vi "Main Tclk.vi"() -> ()   [LabVIEW 2018] (continued)
                          "PID recovered" <- TRUE
                        }
                      }
                    }
                    frame True {
                      w5810 = FALSE
                      n1350 = Divide(x=w5823, y=w5822) -> (x/y=w5821:dbl)
                      n1351 = expression code="x/100"("PID Target (%)") -> (w5816:sgl)
                      n1352 = local write "PID recovered"(w5810) -> ()
                      n1353 = Subtract(x=sgl 1.0, y=w5816) -> (x-y=w5817:sgl)
                      n1354 = Multiply(x=w5821, y=w5817) -> (x*y=w5820:dbl)
                      n1355 = Add(x=w5820, y=w5816) -> (x+y=w5818:dbl)
                      n1356 = Multiply(x=w5818, y=w5811) -> (x*y=w5814:dbl)
                      n1357 = Bundle By Name(cluster=w5812, "FIB PID target"=w5814) -> (w5813:T35)
                      n1358 = local write "Milling para"(w5813) -> ()
                      "Run once" <- w5810
                    }
                  }
                  n1359 = case shown="True" w5786 {
                    frame False {
                    }
                    frame True {
                      n1360 = stacked-sequence {
                        seq-local: [_ w5825 _] -> [_ _ w5860]
                        frame #0 {
                          n1361 = Wait (ms)(milliseconds to wait=u32 2000) -> ()  [unwired: 1 out]
                        }
                        frame #1 {
                          n1362 = local read "Machine Type"() -> (w5826:u8)
                          n1363 = case shown="2" w5826 {
                            tunnel: [w5827 w5835] -> w5825
                            frame 0, Default {
                              n1364 = local read "HV Data Output"() -> (w5831:T18)
                              n1365 = local read "Reheat Parameters"() -> (w5832:T1)
                              n1366 = Unbundle By Name(w5831) -> ("Emission (uA)"=w5833:sgl)
                              n1367 = Unbundle By Name(w5832) -> ("Emission (uA)"=w5834:sgl)
                              n1368 = Subtract(x=w5833, y=w5834) -> (x-y=w5828:sgl)
                              n1369 = Absolute Value(x=w5828) -> (abs(x)=w5829:sgl)
                              n1370 = Greater?(x=0.1 ("y"), y=w5829) -> (0:w5827:bool)
                            }
                            frame 2 {
                              n1371 = stacked-sequence {
                                tunnel: [_ w5859] -> w5835
                                frame #0 {
                                n1372 = local read "FIB HV target matched"() -> (w5837:bool)
                                n1373 = And(x="FIB probe auto min", y=w5837) -> (x .and. y?=w5838:bool)
                                n1374 = case shown="True" w5838 {
                                frame False {
                                }
                                frame True {
                                n1375 = local read "Api"() -> (w5842:refnum<k7>)
                                n1376 = local read "FIB Milling Probe"() -> (w5840:string)
                                n1377 = call "SmartSEM Remote API goto min or max FIB probe current.vi"("Min or Max"="Min", "FIB Probe"=w5840, "Api"=w5842) -> ("Goto probe"=w5841:string)  [unwired: 7 in, 1 out]
                                n1378 = local write "FIB Milling Probe"(w5841) -> ()
                                }
                                }
                                }
                                frame #1 {
                                n1379 = local read "Api"() -> (w5843:refnum<k7>)
                                n1380 = local read "FIB Parameters"() -> (w5858:T19)
                                n1381 = call "SmartSEM Remote API FIB Faraday cup.vi"("Api"=w5843) -> ("FIB Faraday Cup (nA)"=w5856:sgl)  [unwired: 8 in, 2 out]
                                n1382 = call "SmartSEM Remote API get FIB HV data.vi"("Api in"=w5843) -> ("Capella HV Data Output"=w5845:T17)  [unwired: 7 in, 3 out]
                                n1383 = Unbundle By Name(w5858) -> ("FIB probe current"=w5857:sgl)
                                n1384 = Unbundle By Name(w5845) -> ("Emission Target (uA)"=w5847:sgl, "Emission Actual (uA)"=w5846:sgl)
                                n1385 = local read "FIB HV target matched"() -> (w5851:bool)
                                n1386 = Divide(x=w5856, y=w5857) -> (x/y=w5855:sgl)
                                n1387 = Subtract(x=w5847, y=w5846) -> (x-y=w5850:sgl)
                                n1388 = Absolute Value(x=w5850) -> (abs(x)=w5849:sgl)
                                n1389 = In Range and Coerce(upper limit=sgl 1.5 ("y"), x=w5855, lower limit=sgl 0.8 ("y")) -> (In Range?=w5852:bool)  [unwired: 1 out]
                                n1390 = Less?(x=w5849, y=sgl 0.1) -> (x < y?=w5844:bool)
                                n1391 = Compound Arithmetic op=AND(w5851, w5852, w5844) -> (w5859:bool)
                                }
                              }
                            }
                          }
                        }
                        frame #2 {
                          n1392 = case shown="True" w5860 {
                            frame False {
                            }
                            frame True {
                              n1393 = stacked-sequence {
                                frame #0 {
                                w5861 = dbl[] [] ("Re-engage Delta X array")
                                w5862 = 0.0 ("Re-engage X shift")
                                n1394 = local write "Re-engage X shift (um)"(w5862) -> ()
                                n1395 = local write "Re-engage Y shift (um)"(w5862) -> ()
                                n1396 = local write "Re-engage Delta X array"(w5861) -> ()
                                n1397 = local write "Re-engage Delta Y array"(w5861) -> ()
                                n1398 = local write "Re-engage X shift array"(w5861) -> ()
                                n1399 = local write "Re-engage Y shift array"(w5861) -> ()
                                }
                                frame #1 {
                                n1400 = local read "Machine Type"() -> (w5864:u8)
                                n1401 = case shown="2" w5864 {
                                tunnel: [w5865 w5873 w5874] -> w5863
                                frame 0, Default {
                                n1402 = for {
                                N: 10 -> [_]
                                tunnel: [w5870] -> w5867 mode=indexing
                                n1403 = shared-variable ".\\Zeiss Library.lvlib\\Logs"() -> (w5872:sgl[])  [unwired: 1 in, 1 out]
                                n1404 = Index Array(array=w5872, index=0) -> (element=w5870:sgl)
                                n1405 = Wait Until Next ms Multiple(millisecond multiple=u32 10) -> ()  [unwired: 1 out]
                                }
                                n1406 = call-poly <vilib>:"Basic Averaged DC-RMS.vi"("signal in"=w5867) -> ("DC value"=w5866:dbl)  [unwired: 7 in, 3 out]
                                n1407 = To Single Precision Float(number=w5866) -> (single precision float=w5865:sgl)
                                }
                                frame 1 {
                                n1408 = local read "Faraday Cup (nA)"() -> (w5873:sgl)
                                }
                                frame 2 {
                                n1409 = for {
                                N: 10 -> [_]
                                tunnel: [w5879] -> w5876 mode=indexing
                                n1410 = shared-variable ".\\Zeiss Library.lvlib\\Logs"() -> (w5881:sgl[])  [unwired: 1 in, 1 out]
                                n1411 = Index Array(array=w5881, index=0) -> (element=w5879:sgl)
                                n1412 = Wait Until Next ms Multiple(millisecond multiple=u32 10) -> ()  [unwired: 1 out]
                                }
                                n1413 = call-poly <vilib>:"Basic Averaged DC-RMS.vi"("signal in"=w5876) -> ("DC value"=w5875:dbl)  [unwired: 7 in, 3 out]
                                n1414 = To Single Precision Float(number=w5875) -> (single precision float=w5874:sgl)
                                }
                                }
                                n1415 = shared-variable ".\\Zeiss Library.lvlib\\Faraday Cup before mill"(w5863) -> ()  [unwired: 1 in, 1 out]
                                n1416 = local write "Faraday Cup before mill"(w5863) -> ()
                                }
                                frame #2 {
                                w5882 = u8 0 ("Re-engage counts")
                                w5883 = FALSE ("Reheat")
                                n1417 = local write "Re-engage counts"(w5882) -> ()
                                n1418 = local write "Recovered counts"(w5882) -> ()
                                n1419 = local write "Last re-engage count"(w5882) -> ()
                                n1420 = local write "Pause for reheat"(w5883) -> ()
                                n1421 = local write "Mill Manual Pause"(w5883) -> ()
                                n1422 = local write "Reheat from last"(w5883) -> ()
                                }
                                frame #3 {
                                w5885 = TRUE ("Reset WD")
                                n1423 = local read "Alert Settings"() -> (w5884:T36)
                                n1424 = local write "SW error warning armed"(w5885) -> ()
                                n1425 = local write "Auto re-engage"(w5885) -> ()
                                n1426 = local write "3D image paused armed"(w5885) -> ()
                                n1427 = local write "Temperature warning armed"(w5885) -> ()
                                n1428 = local write "Prior Alert Settings"(w5884) -> ()
                                }
                                frame #4 {
                                n1429 = Get Date/Time In Seconds() -> (seconds since 1Jan1904=w5886:timestamp)
                                n1430 = local write "Auto reheat running"(FALSE ("Auto reheat running")) -> ()
                                n1431 = local write "Re-engage time"(w5886) -> ()
                                n1432 = property on="Mill Manual Pause" class="Bool (strict)"("DisabledEnum"=T44."Enabled" ("Disabled")) -> ()  [unwired: 2 in, 2 out]
                                }
                              }
                            }
                          }
                        }
                      }
                    }
                  }
                  n1433 = Compound Arithmetic op=OR(w5790, w5789, w5795) -> (w5796:bool)
                }
                n1434 = case shown="True" w5766 {
                  frame False {
                  }
                  frame True {
                    w5769 = T44."Enabled" ("Disabled")
                    n1435 = property on="Scan x1" class="Bool (strict)"("DisabledEnum"=w5769) -> ()  [unwired: 2 in, 2 out]
                    n1436 = property on="Scan xn" class="Bool (strict)"("DisabledEnum"=w5769) -> ()  [unwired: 2 in, 2 out]
                    n1437 = property on="Start Current DataLog" class="Bool (strict)"("DisabledEnum"=w5769) -> ()  [unwired: 2 in, 2 out]
                    n1438 = property on="Pre image" class="Bool (strict)"("DisabledEnum"=w5769) -> ()  [unwired: 2 in, 2 out]
                    n1439 = property on="Post image" class="Bool (strict)"("DisabledEnum"=w5769) -> ()  [unwired: 2 in, 2 out]
                    n1440 = property on="FIB Imaging" class="Bool (strict)"("DisabledEnum"=w5769) -> ()  [unwired: 2 in, 2 out]
                    n1441 = property on="FIB time lapse" class="Bool (strict)"("DisabledEnum"=w5769) -> ()  [unwired: 2 in, 2 out]
                    n1442 = property on="Reset" class="Bool (strict)"("DisabledEnum"=w5769) -> ()  [unwired: 2 in, 2 out]
                  }
                }
                n1443 = Or(x=w5767, y=w5766) -> (x .or. y?=w5765:bool)
                n1444 = shared-variable "My Computer\\Zeiss Library.lvlib\\Milling Stop"(w5765) -> ()  [unwired: 1 in, 1 out]
                n1445 = shared-variable "My Computer\\Zeiss Library.lvlib\\Milling Resume"(FALSE ("Milling Resume")) -> ()  [unwired: 1 in, 1 out]
              }
              frame #8 {
                w5966 = sgl 0.0 ("Single")
                n1446 = shared-variable ".\\Zeiss Library.lvlib\\Specimen (nA)"() -> (→"Specimen I (nA)":sgl)  [unwired: 1 in, 1 out]
                n1447 = shared-variable ".\\Zeiss Library.lvlib\\Beam Dump 1 (nA)"() -> (→"Beam Dump 1 (nA)":sgl)  [unwired: 1 in, 1 out]
                n1448 = shared-variable ".\\Zeiss Library.lvlib\\Beam Dump 2 (nA)"() -> (→"Beam Dump 2 (nA)":sgl)  [unwired: 1 in, 1 out]
                n1449 = shared-variable ".\\Zeiss Library.lvlib\\Milling I (nA)"() -> (→"Milling I (nA)":sgl)  [unwired: 1 in, 1 out]
                n1450 = shared-variable ".\\Zeiss Library.lvlib\\Milling Z Voltage"() -> (w5947:sgl)  [unwired: 1 in, 1 out]
                "Milling Z voltage (V)" <- w5947
                n1451 = local read "FIB Options"() -> (w5950:T33)
                n1452 = local read "FIB Scan Parameters"() -> (w5948:T32)
                n1453 = local read "Milling para"() -> (w5946:T35)
                n1454 = Unbundle By Name(w5950) -> ("Flip z"=w5965:bool)
                n1455 = Unbundle By Name(w5946) -> ("FIB FOV (um)"=w5958:sgl)
                n1456 = Unbundle By Name(w5946) -> ("X size (um)"=w5944:sgl, "Line milling time (s)"=w5942:sgl, "Lines auto pause"=w5941:u16)
                n1457 = Unbundle By Name(w5948) -> ("Z size (V)"=w5949:dbl)
                n1458 = Negate(x=w5947) -> (-x=w5951:sgl)
                n1459 = Select(t=w5951, s=w5965, f=w5947) -> (s? t:f=w5952:sgl)
                n1460 = Negate(x=w5966) -> (-x=w5967:sgl)
                n1461 = Divide(x=w5952, y=w5949) -> (x/y=w5953:dbl)
                n1462 = Select(t=w5966, s=w5965, f=w5967) -> (s? t:f=w5969:sgl)
                n1463 = Multiply(x=w5953, y=w5958) -> (x*y=w5968:dbl)
                n1464 = Add(x=w5969, y=w5968) -> (x+y=w5970:dbl)
                "FIB profile Y center (um)" <- w5970
                n1465 = call "Milling parameter to trapezoidal shape.vi"("Y location (um)"=w5970, "Milling para"=w5946) -> ("X end"=w5963:dbl, "X start"=w5962:dbl, "X size (um) @ Y"=w5945:dbl)  [unwired: 5 in, 2 out]
                n1466 = expression code="x/2"(w5958) -> (w5959:sgl)
                n1467 = Add(x=w5962, y=w5963) -> (x+y=w5957:dbl)
                n1468 = Divide(x=w5945, y=w5944) -> (x/y=w5943:dbl)
                n1469 = expression code="x/2-30"(w5945) -> (w5955:dbl)
                n1470 = expression code="x/2"(w5957) -> (w5960:dbl)
                n1471 = Compound Arithmetic op=MULTIPLY(w5943, w5942, w5941) -> (→"Milling time (s)":dbl)
                n1472 = Random Number (0-1)() -> (number: 0 to 1=w5954:dbl)
                n1473 = Random Number (0-1)() -> (number: 0 to 1=w5936:dbl)
                n1474 = expression code="(x*2-1)*10"(w5954) -> (w5939:dbl)
                n1475 = Multiply(x=w5959, y=w5960) -> (x*y=w5961:dbl)
                n1476 = In Range and Coerce(upper limit=w5959, x=w5955, lower limit=0.0) -> (coerced(x)=w5938:dbl)  [unwired: 1 out]
                n1477 = Greater?(x=0.5, y=w5936) -> (0:w5934:bool)
                n1478 = Add(x=w5939, y=w5938) -> (x+y=w5937:dbl)
                n1479 = Select(t=1.0 ("f"), s=w5934, f=-1.0) -> (s? t:f=w5931:dbl)
                n1480 = Multiply(x=w5931, y=w5937) -> (x*y=w5930:dbl)
                n1481 = Add(x=w5930, y=w5961) -> (x+y=→"FIB profile X center (um)":dbl)
              }
              frame #9 {
                n1482 = local read "Re-engage counts"() -> (w5983:u8)
                n1483 = local read "Last re-engage count"() -> (w5982:u8)
                n1484 = local read "Low Mag SEM"() -> (w5991:T30)
                n1485 = local read "FIB slice #"() -> (w5989:u32)
                n1486 = local read "Milling para"() -> (w5990:T35)
                n1487 = Unbundle By Name(w5991) -> ("Low mag scan"=w5994:bool, "Prior to main scan"=w5987:bool, "Low mag interval"=w5993:u32)
                n1488 = Select(t=u32 0, s=w5987, f=u32 1 ("t")) -> (s? t:f=w5986:u32)
                n1489 = Unbundle By Name(w5990) -> ("Auto Profile"=w5975:bool)
                n1490 = Subtract(x=w5989, y=w5986) -> (x-y=w5988:u32)
                n1491 = Equal?(x=w5983, y=w5982) -> (x = y?=w5980:bool)
                n1492 = Not Equal To 0?(x=w5982) -> (x != 0?=w5981:bool)
                n1493 = Quotient & Remainder(x=w5988, y=w5993) -> (x-y*floor(x/y)=w5996:u32)  [unwired: 1 out]
                n1494 = And(x=w5980, y=w5981) -> (x .and. y?=w5978:bool)
                n1495 = local read "FIB"() -> (w5992:bool)
                n1496 = Equal To 0?(x=w5996) -> (x = 0?=w5995:bool)
                n1497 = Compound Arithmetic op=AND(w5992, w5994, w5995) -> (w5979:bool)
                n1498 = Or(x=w5978, y=w5979) -> (x .or. y?=w5977:bool)
                n1499 = And(x=w5977, y=w5975) -> (x .and. y?=w5976:bool)
                n1500 = case shown="True" w5976 {
                  frame False {
                  }
                  frame True {
                    n1501 = stacked-sequence {
                      frame #0 {
                        n1502 = local write "FIB Profile"(TRUE ("FIB Profile")) -> ()
                        n1503 = local write "Enable logging"(FALSE ("Enable logging")) -> ()
                        n1504 = Wait (ms)(milliseconds to wait=u32 200) -> ()  [unwired: 1 out]
                      }
                      frame #1 {
                        n1505 = local read "Machine Type"() -> (w6000:u8)
                        n1506 = case shown="2" w6000 {
                          frame 0, Default {
                            w6001 = sgl 90.0 ("UL-Ang")
                            n1507 = local read "FIB profile X center (um)"() -> (w6003:dbl)
                            n1508 = local read "FIB profile Y center (um)"() -> (w6004:dbl)
                            n1509 = local read "HV Data Output"() -> (w6002:T18)
                            n1510 = local read "FIB HW Config"() -> (w6011:T23)
                            n1511 = local read "FIB Options"() -> (w6012:T33)
                            n1512 = local read "Milling para"() -> (w6008:T35)
                            n1513 = local read "FIB Scan Parameters"() -> (w6009:T32)
                            n1514 = local read "Parameter Names"() -> (w6015:string[])
                            n1515 = Bundle By Name(cluster=w6009, "Frame line rampdown ratio"=0.0, "Oversampling"=u16 5) -> (w6013:T32)
                            n1516 = Bundle By Name(cluster=w6008, "X size (um)"=sgl 0.1, "Z size (um)"=sgl 10.0 ("Y size (um)"), "X center (um)"=w6003, "Z center (um)"=w6004, "UL-Ang"=w6001, "UR-Ang"=w6001) -> (w6007:T35)
                            n1517 = local read "Active logging channels"() -> (w6014:string)
                            n1518 = local write "Status message"("Scanning FIB vertically to obtain beam profile" ("Status message")) -> ()
                            n1519 = call "FIB profile.vi"("HV Data Output"=w6002, "Parameter Names"=w6015, "Active logging channels"=w6014, "Scan Para"=w6013, "Milling para"=w6007, "Options"=w6012, "HW Config"=w6011) -> ("Measurements"=w6017:dbl[][])  [unwired: 2 in, 2 out]
                            n1520 = local write "Measurements"(w6017) -> ()
                          }
                          frame 2 {
                            w6019 = sgl 90.0 ("UL-Ang")
                            n1521 = local read "FIB profile X center (um)"() -> (w6021:dbl)
                            n1522 = local read "FIB profile Y center (um)"() -> (w6022:dbl)
                            n1523 = local read "FIB HW Config"() -> (w6029:T23)
                            n1524 = local read "FIB Options"() -> (w6030:T33)
                            n1525 = local read "Milling para"() -> (w6026:T35)
                            n1526 = local read "FIB Scan Parameters"() -> (w6027:T32)
                            n1527 = local read "Parameter Names"() -> (w6033:string[])
                            n1528 = local read "Capella HV Data Output"() -> (w6020:T17)
                            n1529 = Bundle By Name(cluster=w6027, "Frame line rampdown ratio"=0.0, "Oversampling"=u16 5) -> (w6031:T32)
                            n1530 = local read "Active logging channels"() -> (w6032:string)
                            n1531 = Bundle By Name(cluster=w6026, "X size (um)"=sgl 0.1, "Z size (um)"=sgl 10.0 ("Y size (um)"), "X center (um)"=w6021, "Z center (um)"=w6022, "UL-Ang"=w6019, "UR-Ang"=w6019) -> (w6025:T35)
                            n1532 = local write "Status message"("Scanning FIB vertically to obtain beam profile" ("Status message")) -> ()
                            n1533 = call "FIB profile.vi"("Capella HV Data Output"=w6020, "Parameter Names"=w6033, "Active logging channels"=w6032, "Scan Para"=w6031, "Milling para"=w6025, "Options"=w6030, "HW Config"=w6029) -> ("Measurements"=w6035:dbl[][])  [unwired: 2 in, 2 out]
                            n1534 = local write "Measurements"(w6035) -> ()
                          }
                        }
                      }
                      frame #2 {
                        n1535 = local write "FIB Profile"(FALSE ("FIB Profile")) -> ()
                        n1536 = local write "Enable logging"(TRUE ("Enable logging")) -> ()
                      }
                    }
                  }
                }
              }
              frame #10 {
                n1537 = local read "FIB"() -> (w6045:bool)
                n1538 = local read "Auto re-engage"() -> (w6041:bool)
                n1539 = local read "Milling para"() -> (w6043:T35)
                n1540 = local read "Machine Type"() -> (w6042:u8)
                n1541 = case shown="True" w6045 {
                  frame False {
                  }
                  frame True {
                    n1542 = local read "Post #1up"() -> (w6066:tag)
                    n1543 = local read "Post #1down"() -> (w6068:tag)
                    n1544 = local read "Post #2up"() -> (w6067:tag)
                    n1545 = local read "Post #2down"() -> (w6069:tag)
                    n1546 = call "SEM shutter.vi"("Shutter close"=FALSE, "Shutter AO4"=w6069, "Shutter AO3"=w6067, "Shutter AO2"=w6068, "Shutter AO1"=w6066) -> ()  [unwired: 6 in, 1 out]
                  }
                }
                n1547 = Unbundle By Name(w6043) -> ("FIB PID measured"=w6044:u8)
                n1548 = case shown="0" w6044 {
                  tunnel: w6042 -> [w6056 _ w6060 _]
                  tunnel: [w6055 0.5 ("Minimum half range") w6061 0.5 ("Minimum half range")] -> w6040
                  frame 0 {
                    n1549 = case shown="0, Default" w6056 {
                      tunnel: [0.5 ("Minimum half range") 0.8 ("Minimum half range")] -> w6055
                      frame 0, Default {
                      }
                      frame 2 {
                      }
                    }
                  }
                  frame 1 {
                  }
                  frame 2 {
                    n1550 = case shown="2" w6060 {
                      tunnel: [0.3 ("Minimum half range") 0.6 ("Minimum half range")] -> w6061
                      frame 0, Default {
                      }
                      frame 2 {
                      }
                    }
                  }
                  frame 3, Default {
                  }
                }
                n1551 = case shown="True" w6041 {
                  tunnel: [w6046 w6047] -> w6039
                  tunnel: w6040 -> [w6046 w6048]
                  frame False {
                  }
                  frame True {
                    n1552 = local read "Re-engage counts"() -> (w6049:u8)
                    n1553 = case shown="1" w6049 {
                      tunnel: [w6050 w6051 w6053] -> w6047
                      tunnel: w6048 -> [w6050 w6052 w6054]
                      frame 0, Default {
                      }
                      frame 1 {
                        n1554 = expression code="x*4"(w6052) -> (w6051:dbl)
                      }
                      frame 2 {
                        n1555 = expression code="x*2"(w6054) -> (w6053:dbl)
                      }
                    }
                  }
                }
                "FIB CL control band" <- w6039
              }
              frame #11 {
                n1556 = local read "Low Mag SEM"() -> (w6072:T30)
                n1557 = local read "FIB slice #"() -> (w6071:u32)
                n1558 = Unbundle By Name(w6072) -> ("Low mag scan"=w6075:bool, "Prior to main scan"=w6074:bool, "Low mag interval"=w6070:u32)
                n1559 = Quotient & Remainder(x=w6071, y=w6070) -> (x-y*floor(x/y)=w6077:u32)  [unwired: 1 out]
                n1560 = local read "FIB"() -> (w6073:bool)
                n1561 = Equal To 0?(x=w6077) -> (x = 0?=w6076:bool)
                n1562 = Compound Arithmetic op=AND(w6073, w6075, w6074, w6076) -> (w6078:bool)
                n1563 = case shown="True" w6078 {
                  frame False {
                    n1564 = local write "Low Mag SEM on"(FALSE ("Mid Mag SEM on")) -> ()
                    n1565 = local write "LM overhead"(u32 0 ("LM overhead")) -> ()
                  }
                  frame True {
                    n1566 = stacked-sequence {
                      seq-local: [w6084 _] -> [_ w6093]
                      frame #0 {
                        n1567 = local read "LM SEM scan time"() -> (w6083:dbl)
                        n1568 = local read "Tiled scan inputs"() -> (w6085:T6)
                        n1569 = local read "SEM HW Config"() -> (w6086:T9)
                        n1570 = local read "Detector Information"() -> (w6087:T8)
                        n1571 = local read "SEM Scan Parameters"() -> (w6088:T26)
                        n1572 = local read "SEM Options"() -> (w6089:T27)
                        n1573 = local read "Focus Index Options"() -> (w6081:T28)
                        n1574 = local read "File Information"() -> (w6090:T31)
                        n1575 = local read "Milling para"() -> (w6091:T35)
                        n1576 = Bundle By Name(cluster=w6085, "HW Config"=w6086, "Det Info"=w6087, "SEM Scan Parameters"=w6088, "SEM Options"=w6089, "Focus Index Options"=w6081, "File Information"=w6090, "Milling para"=w6091) -> (w6084:T6)
                        n1577 = expression code="x+10"(w6083) -> (w6082:dbl)
                        n1578 = local write "LM overhead"(w6082) -> ()
                      }
                      frame #1 {
                        w6094 = FALSE ("GetInfo")
                        n1579 = local read "SEM Low Mag Scan Parameters"() -> (w6097:T5)
                        n1580 = local read "File Information"() -> (w6098:T31)
                        n1581 = Unbundle By Name(w6098) -> ("File path"=w6100:path)
                        n1582 = local write "Status message"("SEM Low Mag Scan" ("Status message")) -> ()
                        n1583 = Build Path(base path=w6100, name or relative path="Low Mag Scans\\") -> (appended path=w6101:path)
                        n1584 = Bundle By Name(cluster=w6093, "SEM Options.GetInfo"=w6094, "SEM Options.PNG only"=TRUE ("PNG only"), "SEM Options.Upload"=w6094, "SEM Scan Parameters"=w6097, "File Information.File path"=w6101) -> (w6096:T6)
                        n1585 = call "2D scan tiled.vi"("Tiled scan inputs"=w6096) -> ()  [unwired: 5 in, 6 out]
                        "Low Mag SEM on" <- TRUE ("Mid Mag SEM on")
                      }
                    }
                  }
                }
              }
              frame #12 {
                n1586 = local read "Mid Mag SEM"() -> (w6114:T29)
                n1587 = local read "FIB slice #"() -> (w6113:u32)
                n1588 = Subtract(x=w6113, y=u32 2) -> (x-y=w6104:u32)
                n1589 = Unbundle By Name(w6114) -> ("Mid mag scan"=w6111:bool, "Prior to main scan"=w6118:bool, "Mid mag interval"=w6103:u32)
                n1590 = Equal?(x=u32 1 ("y"), y=w6103) -> (x = y?=w6105:bool)
                n1591 = case shown="False" w6105 {
                  tunnel: [w6122 w6125] -> w6110
                  tunnel: [w6121 w6125] -> w6109
                  tunnel: [w6119 w6125] -> w6107
                  frame False {
                    n1592 = local read "Auto Focus"() -> (w6124:bool)
                    n1593 = local read "Auto Stig"() -> (w6123:bool)
                    n1594 = local read "Auto Align"() -> (w6120:bool)
                    n1595 = Not(x=w6124) -> (.not. x?=w6121:bool)
                    n1596 = Not(x=w6123) -> (.not. x?=w6122:bool)
                    n1597 = Not(x=w6120) -> (.not. x?=w6119:bool)
                  }
                  frame True {
                    w6125 = TRUE
                  }
                }
                n1598 = Quotient & Remainder(x=w6104, y=w6103) -> (x-y*floor(x/y)=w6116:u32)  [unwired: 1 out]
                n1599 = local read "FIB"() -> (w6112:bool)
                n1600 = Equal To 0?(x=w6116) -> (x = 0?=w6117:bool)
                n1601 = Compound Arithmetic op=AND(w6112, w6109, w6110, w6107, w6111, w6118, w6117) -> (w6115:bool)
                n1602 = case shown="True" w6115 {
                  frame False {
                    n1603 = local write "Mid Mag SEM on"(FALSE ("Mid Mag SEM on")) -> ()
                    n1604 = local write "MM overhead"(u32 0 ("MM overhead")) -> ()
                  }
                  frame True {
                    n1605 = stacked-sequence {
                      seq-local: [w6131 _] -> [_ w6139]
                      frame #0 {
                        n1606 = local read "Tiled scan inputs"() -> (w6132:T6)
                        n1607 = local read "SEM HW Config"() -> (w6133:T9)
                        n1608 = local read "Detector Information"() -> (w6134:T8)
                        n1609 = local read "SEM Scan Parameters"() -> (w6135:T26)
                        n1610 = local read "SEM Options"() -> (w6136:T27)
                        n1611 = local read "Focus Index Options"() -> (w6128:T28)
                        n1612 = local read "File Information"() -> (w6137:T31)
                        n1613 = local read "Milling para"() -> (w6138:T35)
                        n1614 = local read "MM SEM scan time"() -> (w6129:dbl)
                        n1615 = Bundle By Name(cluster=w6132, "HW Config"=w6133, "Det Info"=w6134, "SEM Scan Parameters"=w6135, "SEM Options"=w6136, "Focus Index Options"=w6128, "File Information"=w6137, "Milling para"=w6138) -> (w6131:T6)
                        n1616 = expression code="x+10"(w6129) -> (w6130:dbl)
                        n1617 = local write "MM overhead"(w6130) -> ()
                      }
                      frame #1 {
                        w6146 = FALSE ("GetInfo")
                        n1618 = local read "SEM Mid Mag Scan Parameters"() -> (w6144:T5)
                        n1619 = local read "File Information"() -> (w6143:T31)
                        n1620 = Unbundle By Name(w6143) -> ("File path"=w6141:path)
                        n1621 = local write "Status message"("SEM Mid Mag Scan" ("Status message")) -> ()
                        n1622 = Build Path(base path=w6141, name or relative path="Mid Mag Scans\\") -> (appended path=w6140:path)
                        n1623 = Bundle By Name(cluster=w6139, "SEM Options.GetInfo"=w6146, "SEM Options.PNG only"=w6146, "SEM Options.Upload"=w6146, "SEM Scan Parameters"=w6144, "File Information.File path"=w6140) -> (w6145:T6)
                        n1624 = call "2D scan tiled.vi"("Tiled scan inputs"=w6145) -> ()  [unwired: 5 in, 6 out]
                        "Mid Mag SEM on" <- TRUE ("Mid Mag SEM on")
                      }
                    }
                  }
                }
              }
              frame #13 {
                n1625 = local read "Auto re-engage"() -> (w6149:bool)
                n1626 = case shown="False" w6149 {
                  frame False {
                    n1627 = local read "Auto Align"() -> (w6151:bool)
                    n1628 = local read "Auto Focus"() -> (w6153:bool)
                    n1629 = local read "Auto Stig"() -> (w6152:bool)
                    n1630 = local read "Re-engage counts"() -> (w6157:u8)
                    n1631 = local read "Last re-engage count"() -> (w6156:u8)
                    n1632 = Build Array(w6153, w6152, w6151) -> (w6154:bool[])
                    n1633 = Equal?(x=w6157, y=w6156) -> (x = y?=w6155:bool)
                    n1634 = Boolean Array To Number(Boolean array=w6154) -> (number=w6150:u32)
                    n1635 = case shown="6" w6150 {
                      frame 0, Default {
                      }
                      frame 3 {
                        n1636 = local write "Auto Stig"(FALSE ("Auto Focus")) -> ()
                      }
                      frame 5 {
                        n1637 = local write "Auto Align"(FALSE ("Auto Focus")) -> ()
                      }
                      frame 6 {
                        n1638 = local write "Auto Align"(FALSE ("Auto Focus")) -> ()
                      }
                      frame 7 {
                        w6162 = FALSE ("Auto Focus")
                        n1639 = local write "Auto Stig"(w6162) -> ()
                        n1640 = local write "Auto Align"(w6162) -> ()
                      }
                    }
                    n1641 = case shown="False" w6155 {
                      tunnel: [w6164 w6165] -> w6158
                      tunnel: w6157 -> [w6163 _]
                      frame False {
                        n1642 = Increment(x=w6163) -> (x+1=w6164:u8)
                      }
                      frame True {
                        w6165 = u8 0
                        n1643 = local write "Last re-engage count"(w6165) -> ()
                      }
                    }
                    n1644 = local write "Re-engage counts"(w6158) -> ()
                  }
                  frame True {
                    w6168 = T44."Enabled" ("Disabled")
                    w6169 = T44."Disabled and Grayed Out" ("Disabled")
                    w6170 = u8 0 ("AF Count")
                    w6167 = 0.0 ("f")
                    w6172 = FALSE ("Auto Focus")
                    n1645 = local write "Auto Focus"(w6172) -> ()
                    n1646 = local write "Auto Stig"(w6172) -> ()
                    n1647 = local write "Auto Align"(w6172) -> ()
                    n1648 = local read "Focus Index"() -> (w6202:sgl)
                    n1649 = local read "Pre-reheat FI"() -> (w6203:dbl)
                    n1650 = local read "Pre-reheat X center (um)"() -> (w6189:dbl)
                    n1651 = local read "Re-engage X shift (um)"() -> (w6177:dbl)
                    n1652 = local read "Pre-reheat Y center (um)"() -> (w6204:dbl)
                    n1653 = local read "Re-engage Y shift (um)"() -> (w6180:dbl)
                    n1654 = local read "Pre-reheat Y stig"() -> (w6171:sgl[][])
                    n1655 = local read "FIB-SEM Angle"() -> (w6174:dbl)
                    n1656 = expression code="x*0.9"(w6203) -> (w6201:dbl)
                    n1657 = expression code="cos(x*pi/180)"(w6174) -> (w6173:dbl)
                    n1658 = local write "AF Count"(w6170) -> ()
                    n1659 = local write "AS Count"(w6170) -> ()
                    n1660 = local write "AA Count"(w6170) -> ()
                    n1661 = local read "Re-engage counts"() -> (w6182:u8)
                    n1662 = local read "Recovered counts"() -> (w6195:u8)
                    n1663 = local write "Re-engage cancelled"("Cancel Auto re-engage") -> ()
                    n1664 = Greater Or Equal?(x=w6202, y=w6201) -> (x >= y?=w6199:bool)
                    n1665 = Power Of X(1:w6180, 2:"b") -> (0:w6186:dbl)
                    n1666 = Select(t=u8 1, s=w6199, f=u8 0) -> (s? t:f=w6196:u8)
                    n1667 = Compound Arithmetic op=MULTIPLY(w6186, "a", w6173) -> (w6184:dbl)
                    "Re-engage Y stig shift" <- w6184
                    n1668 = Increment(x=w6182) -> (x+1=w6181:u8)
                    n1669 = Add(x=w6196, y=w6195) -> (x+y=w6183:u8)
                    n1670 = Not(x="Cancel Auto re-engage") -> (.not. x?=w6200:bool)
                    n1671 = local write "Re-engage counts"(w6181) -> ()
                    n1672 = Less Or Equal?(x=w6183, y=u8 11) -> (x <= y?=w6193:bool)
                    n1673 = local write "Recovered counts"(w6183) -> ()
                    n1674 = And(x=w6193, y=w6200) -> (x .and. y?=w6191:bool)
                    n1675 = Select(t=w6177, s=w6191, f=w6167) -> (s? t:f=w6190:dbl)
                    n1676 = Select(t=w6180, s=w6191, f=w6167) -> (s? t:f=w6192:dbl)
                    n1677 = Select(t=w6184, s=w6191, f=w6167) -> ()  [unwired: 1 out]
                    n1678 = Add(x=w6189, y=w6190) -> (x+y=w6188:dbl)
                    n1679 = Add(x=w6204, y=w6192) -> (x+y=w6207:dbl)
                    n1680 = Add(x=w6171, y=w6167) -> (x+y=w6205:dbl[][])
                    n1681 = local write "Auto re-engage"(w6191) -> ()
                    n1682 = case shown="False" w6191 {
                      tunnel: w6181 -> [w6212 _]
                      frame False {
                        w6209 = T44."Enabled" ("Disabled")
                        n1683 = Increment(x=w6212) -> (x+1=w6211:u8)
                        n1684 = local read "Prior Alert Settings"() -> (w6210:T2)
                        n1685 = local write "Last re-engage count"(w6211) -> ()
                        n1686 = local write "Recovered counts"(u8 0 ("Recovered counts")) -> ()
                        n1687 = property on="Pause for reheat" class="Bool (strict)"("DisabledEnum"=T44."Enabled" ("Disabled")) -> ()  [unwired: 2 in, 2 out]
                        n1688 = local write "Alert Settings"(w6210) -> ()
                        n1689 = local write "Cancel Auto re-engage"(FALSE ("Cancel Auto re-engage")) -> ()
                        n1690 = property on="Auto Focus" class="Bool (strict)"("DisabledEnum"=w6209) -> ()  [unwired: 2 in, 2 out]
                        n1691 = property on="Auto Stig" class="Bool (strict)"("DisabledEnum"=w6209) -> ()  [unwired: 2 in, 2 out]
                        n1692 = property on="Auto Align" class="Bool (strict)"("DisabledEnum"=w6209) -> ()  [unwired: 2 in, 2 out]
                      }
                      frame True {
                      }
                    }
                    n1693 = local read "SEM Scan Parameters"() -> (w6208:T26)
                    n1694 = Bundle By Name(cluster=w6208, "X center (um)"=w6188, "Y center (um)"=w6207, "Y stig"=w6205) -> (w6206:T26)
                    n1695 = local write "SEM Scan Parameters"(w6206) -> ()
                    n1696 = property on="Auto Focus" class="Bool (strict)"("DisabledEnum"=w6169) -> ()  [unwired: 2 in, 2 out]
                    n1697 = property on="Auto Stig" class="Bool (strict)"("DisabledEnum"=w6169) -> ()  [unwired: 2 in, 2 out]
                    n1698 = property on="Auto Align" class="Bool (strict)"("DisabledEnum"=w6169) -> ()  [unwired: 2 in, 2 out]
                    n1699 = local read "Re-engage X shift array"() -> (w6176:dbl[])
                    n1700 = local read "Re-engage Y shift array"() -> (w6179:dbl[])
                    n1701 = property on="AF Steps" class="DigNum (strict)"("DisabledEnum"=w6168) -> ()  [unwired: 2 in, 2 out]
                    n1702 = property on="AS Steps" class="DigNum (strict)"("DisabledEnum"=w6168) -> ()  [unwired: 2 in, 2 out]
                    n1703 = property on="AA Steps" class="DigNum (strict)"("DisabledEnum"=w6168) -> ()  [unwired: 2 in, 2 out]
                    n1704 = Build Array (concatenate)(w6176, w6177) -> (w6175:dbl[])
                    n1705 = Build Array (concatenate)(w6179, w6180) -> (w6178:dbl[])
                    n1706 = local write "Re-engage X shift array"(w6175) -> ()
                    n1707 = local write "Re-engage Y shift array"(w6178) -> ()
                  }
                }
              }
              frame #14 {
                n1708 = case shown="False" "Auto Focus" {
                  frame False {
                    n1709 = local read "WD array tiled"() -> (w6218:sgl[][][])
                    n1710 = local read "Auto Stig"() -> (w6223:bool)
                    n1711 = local read "Auto Align"() -> (w6222:bool)
                    n1712 = Not(x=w6223) -> (.not. x?=w6220:bool)
                    n1713 = Not(x=w6222) -> (.not. x?=w6219:bool)
                    n1714 = Empty Array?(array=w6218) -> (empty?=w6217:bool)
                    n1715 = Compound Arithmetic op=AND(w6217, w6220, w6219) -> (w6221:bool)
                    n1716 = case shown="False" w6217 {
                      frame False {
                        n1717 = property on="Auto Focus" class="Bool (strict)"("DisabledEnum"=T44."Disabled and Grayed Out" ("Disabled")) -> ()  [unwired: 2 in, 2 out]
                      }
                      frame True {
                      }
                    }
                    n1718 = case shown="True" w6221 {
                      frame False {
                      }
                      frame True {
                        w6224 = T44."Enabled" ("Disabled")
                        n1719 = property on="Auto Stig" class="Bool (strict)"("DisabledEnum"=w6224) -> ()  [unwired: 2 in, 2 out]
                        n1720 = property on="Auto Align" class="Bool (strict)"("DisabledEnum"=w6224) -> ()  [unwired: 2 in, 2 out]
                      }
                    }
                  }
                  frame True {
                    w6235 = T44."Disabled and Grayed Out" ("Disabled")
                    n1721 = local read "SEM Scan Parameters"() -> (w6233:T26)
                    n1722 = local read "AF Count"() -> (w6230:u8)
                    n1723 = Increment(x=w6230) -> (x+1=w6234:u8)
                    n1724 = Equal To 0?(x=w6230) -> (x = 0?=w6229:bool)
                    n1725 = local write "AF Count"(w6234) -> ()
                    n1726 = property on="Auto Stig" class="Bool (strict)"("DisabledEnum"=w6235) -> ()  [unwired: 2 in, 2 out]
                    n1727 = property on="X Grids" class="Arr (strict)"("DisabledEnum"=w6235) -> ()  [unwired: 2 in, 2 out]
                    n1728 = property on="Primary X index" class="Arr (strict)"("DisabledEnum"=w6235) -> ()  [unwired: 2 in, 2 out]
                    n1729 = Unbundle By Name(w6233) -> ("Y tiles"=w6232:u8, "X tiles"=w6231:u8)
                    n1730 = property on="Auto Align" class="Bool (strict)"("DisabledEnum"=w6235) -> ()  [unwired: 2 in, 2 out]
                    n1731 = case shown="True" w6229 {
                      tunnel: w6232 -> [_ w6241]
                      tunnel: w6231 -> [_ w6242]
                      frame False {
                      }
                      frame True {
                        n1732 = Initialize Array(FALSE ("ASX Success"), w6241, w6242) -> (w6246:bool[][])
                        n1733 = Initialize Array(u8 0 ("Skip Steps"), w6241, w6242) -> (w6243:u8[][])
                        n1734 = local write "Skip Steps tiled"(w6243) -> ()
                        n1735 = local write "AF Success tiled"(w6246) -> ()
                        n1736 = local write "Image Tabs"(T37."Auto Focus / Stig / Align" ("Image Tabs")) -> ()
                      }
                    }
                    n1737 = property on="Y Grids" class="Arr (strict)"("DisabledEnum"=w6235) -> ()  [unwired: 2 in, 2 out]
                    n1738 = property on="Primary Y index" class="Arr (strict)"("DisabledEnum"=w6235) -> ()  [unwired: 2 in, 2 out]
                    n1739 = property on="Keep aspect ratio" class="Bool (strict)"("DisabledEnum"=w6235) -> ()  [unwired: 2 in, 2 out]
                    n1740 = local read "Focus Index Options"() -> (w6228:T28)
                    n1741 = Unbundle By Name(w6228) -> ("Y Grids"=w6227:u8[][])
                    n1742 = Array Max & Min(array=w6227) -> (max value=w6226:u8)  [unwired: 3 out]
                    n1743 = Greater Or Equal?(x=w6226, y=u8 2) -> (x >= y?=w6239:bool)
                    n1744 = Select(t=T44."Enabled" ("Disabled"), s=w6239, f=T44."Disabled and Grayed Out" ("Disabled")) -> (s? t:f=w6236:T44)
                    n1745 = property on="Slope tiled" class="Arr (strict)"("DisabledEnum"=w6236) -> ()  [unwired: 2 in, 2 out]
                    n1746 = property on="Dynamic Focus" class="XYGraph (strict)"("DisabledEnum"=w6236) -> ()  [unwired: 2 in, 2 out]
                  }
                }
              }
              frame #15 {
                n1747 = case shown="False" "Auto Stig" {
                  frame False {
                    n1748 = local read "StigX array tiled"() -> (w6284:sgl[][][])
                    n1749 = local read "StigY array tiled"() -> (w6285:sgl[][][])
                    n1750 = local read "Auto Focus"() -> (w6288:bool)
                    n1751 = local read "Auto Align"() -> (w6289:bool)
                    n1752 = Empty Array?(array=w6284) -> (empty?=w6283:bool)
                    n1753 = Empty Array?(array=w6285) -> (empty?=w6282:bool)
                    n1754 = local write "Stig Options"(enum16{"Defaut", "Stig X", "Stig Y"}."Defaut" ("Stig Options")) -> ()
                    n1755 = Not(x=w6288) -> (.not. x?=w6290:bool)
                    n1756 = Not(x=w6289) -> (.not. x?=w6291:bool)
                    n1757 = And(x=w6283, y=w6282) -> (x .and. y?=w6286:bool)
                    n1758 = Compound Arithmetic op=AND(w6286, w6290, w6291) -> (w6287:bool)
                    n1759 = case shown="False" w6286 {
                      frame False {
                        n1760 = property on="Auto Stig" class="Bool (strict)"("DisabledEnum"=T44."Disabled and Grayed Out" ("Disabled")) -> ()  [unwired: 2 in, 2 out]
                      }
                      frame True {
                      }
                    }
                    n1761 = case shown="True" w6287 {
                      frame False {
                      }
                      frame True {
                        w6293 = T44."Enabled" ("Disabled")
                        n1762 = property on="Auto Focus" class="Bool (strict)"("DisabledEnum"=w6293) -> ()  [unwired: 2 in, 2 out]
                        n1763 = property on="Auto Align" class="Bool (strict)"("DisabledEnum"=w6293) -> ()  [unwired: 2 in, 2 out]
                      }
                    }
                  }
                  frame True {
                    w6301 = T44."Disabled and Grayed Out" ("Disabled")
                    n1764 = local read "SEM Scan Parameters"() -> (w6299:T26)
                    n1765 = local read "AS Count"() -> (w6296:u8)
                    n1766 = local read "Stig Options"() -> (w6305:enum16{"Defaut", "Stig X", "Stig Y"})
                    n1767 = Increment(x=w6296) -> (x+1=w6300:u8)
                    n1768 = Equal To 0?(x=w6296) -> (x = 0?=w6295:bool)
                    n1769 = local write "AS Count"(w6300) -> ()
                    n1770 = Unbundle By Name(w6299) -> ("Y tiles"=w6298:u8, "X tiles"=w6297:u8)
                    n1771 = Equal?(x=w6305, y=enum16{"Defaut", "Stig X", "Stig Y"}."Defaut" ("Stig Options")) -> (x = y?=w6302:bool)
                    n1772 = property on="Auto Focus" class="Bool (strict)"("DisabledEnum"=w6301) -> ()  [unwired: 2 in, 2 out]
                    n1773 = And(x=w6295, y=w6302) -> (x .and. y?=w6303:bool)
                    n1774 = case shown="True" w6303 {
                      tunnel: w6298 -> [_ w6308]
                      tunnel: w6297 -> [_ w6307]
                      frame False {
                      }
                      frame True {
                        n1775 = Initialize Array(FALSE ("ASX Success"), w6308, w6307) -> (w6311:bool[][])
                        n1776 = Initialize Array(u8 0 ("Skip Steps"), w6308, w6307) -> (w6306:u8[][])
                        n1777 = local write "ASX Success tiled"(w6311) -> ()
                        n1778 = local write "ASY Success tiled"(w6311) -> ()
                        n1779 = local write "Skip Steps tiled"(w6306) -> ()
                        n1780 = local write "Stig Options"(enum16{"Defaut", "Stig X", "Stig Y"}."Stig X" ("Stig Options")) -> ()
                        n1781 = local write "Image Tabs"(T37."Auto Focus / Stig / Align" ("Image Tabs")) -> ()
                      }
                    }
                    n1782 = property on="Auto Align" class="Bool (strict)"("DisabledEnum"=w6301) -> ()  [unwired: 2 in, 2 out]
                  }
                }
                n1783 = case shown="True" "Auto Align" {
